vi "HasNext.vi"(8 "error in (no error)":errorcluster, 11 "Iterator":refnum<class "Iterator.lvclass">) -> (0 "error out":errorcluster, 2 "HasNext?(False)":bool, 3 "Iterator out":refnum<class "Iterator.lvclass">)   [LabVIEW 2015, in "Iterator.lvclass"]
uses:
  Iterator.lvclass
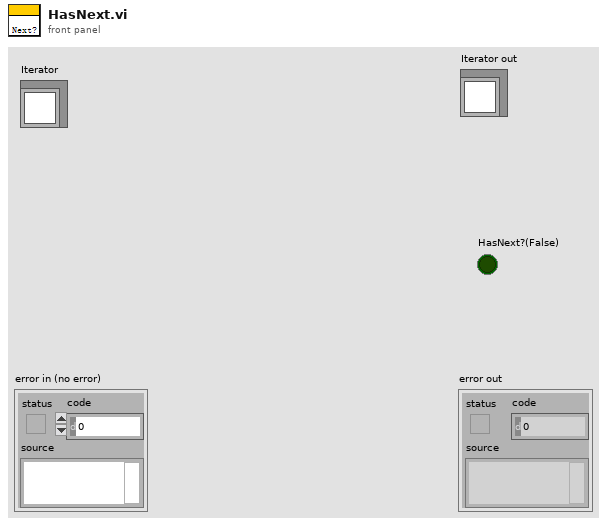
[diagram p1: front panel]
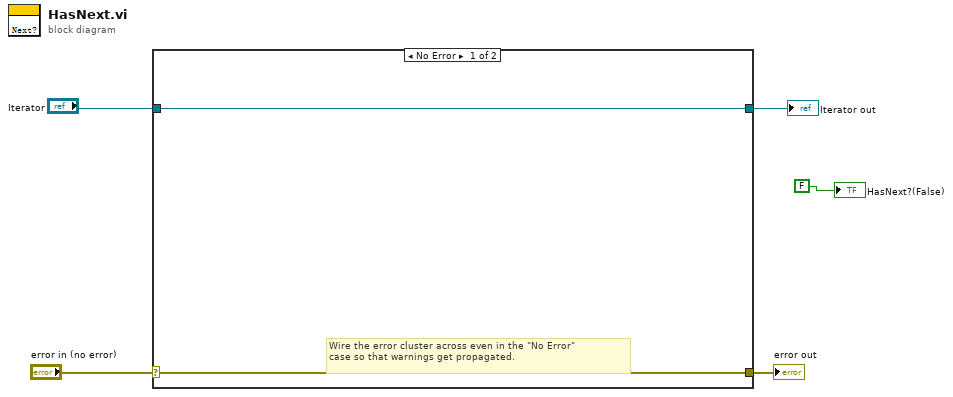
[diagram p0: block diagram]
diagram:
  n1 = case shown="No Error" "error in (no error)" {
    selector: "error in (no error)" -> [w6 w9]
    tunnel: [w6 w9] -> w4
    tunnel: [w7 w8] -> w1
    tunnel: "Iterator" -> [w7 w8]
    frame No Error {
      # "Wire the error cluster across even in the \"No Error\"\ncase so that warnings get propagated."
    }
    frame Error {
    }
  }
  "error out" <- w4
  "Iterator out" <- w1
  "HasNext?(False)" <- FALSE
